vi "writeToXML.vi"(8 "error in (no error)":errorcluster, 10 "ClassLabel":string, 11 "MccRotStop in":refnum<class "MccRotStop.lvclass">) -> (0 "error out":errorcluster, 2 "XMLout":string, 3 "MccRotStop out":refnum<class "MccRotStop.lvclass">)   [LabVIEW 2022 SP3, in "TCSDataDefinitions.lvlib" / "TCSMountControlCommand.lvlib" / "CommandsForRotatorAxis.lvlib" / "MccRotStop.lvclass"]
uses:
  MccRotStop.lvclass
  CommandsForRotatorAxis.lvclass
  <userlib>/Common/XML/XMLGenerator/XMLGenerator.lvclass
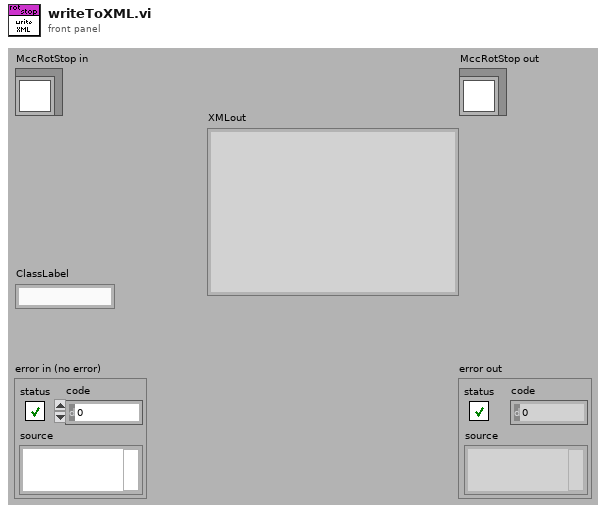
[diagram p1: front panel]
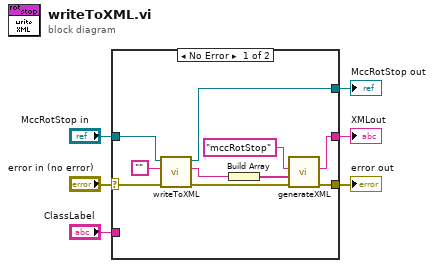
[diagram p0: block diagram]
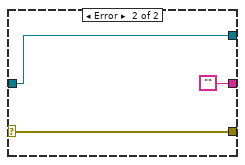
[diagram p2: hidden frame]
diagram:
  n1 = case shown="No Error" "error in (no error)" {
    selector: "error in (no error)" -> [w9 w19]
    tunnel: [w8 w19] -> w5
    tunnel: [w10 w18] -> w3
    tunnel: "MccRotStop in" -> [w11 w18]
    tunnel: [w7 ""] -> w2
    tunnel: "ClassLabel" -> [_ _]
    frame No Error {
      n2 = call-parent "writeToXML.vi"("error in (no error)"=w9, "ClassLabel"="", "CommandsForRotatorAxis in"=w11) -> ("error out"=w12:errorcluster, "XMLout"=w15:string, "CommandsForRotatorAxis out"=w10:refnum<class "MccRotStop.lvclass">)  [unwired: 6 in]
      n3 = Build Array(w15) -> (w14:string[])
      n4 = call <userlib>:"generateXML.vi"("error in"=w12, "childrenXML"=w14, "elementName"="mccRotStop" ("Class Label")) -> ("error out"=w8:errorcluster, "XML out"=w7:string)  [unwired: 6 in, 1 out]
    }
    frame Error {
    }
  }
  "error out" <- w5
  "MccRotStop out" <- w3
  "XMLout" <- w2
